vi "Build SendInput Struct.vi"(8 "error in (no error)":errorcluster, 10 "Data":u8[](array[numeric]), 11 "type":T1) -> (0 "error out":errorcluster, 3 "INPUT":u8[](array[numeric]))   [LabVIEW 2020, in "MacroAssert.lvlib" / "Win Util.lvlib"]
uses:
  Win Util.lvlib
  Input Type.ctl
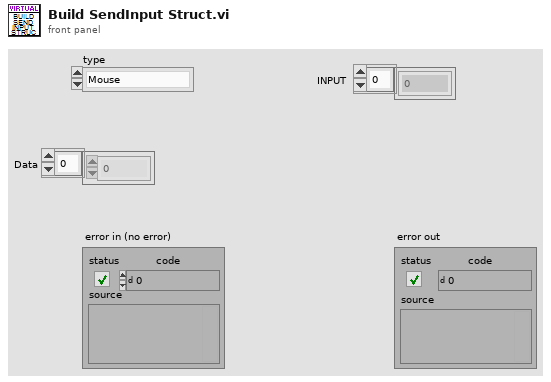
[diagram p1: front panel]
types:
  T1 = typedef "MacroAssert.lvlib/Win Util.lvlib/Input Type.ctl" = enum16{"Mouse", "Keyboard", "Hardware"}
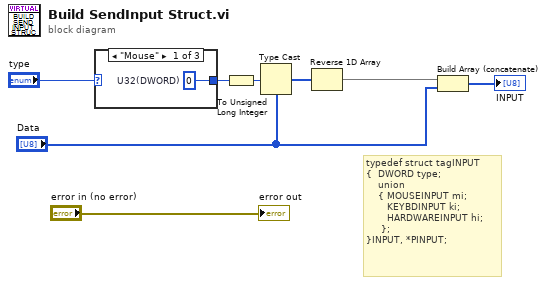
[diagram p0: block diagram]
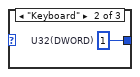
[diagram p2: hidden frame]
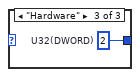
[diagram p3: hidden frame]
diagram:
  # "typedef struct tagINPUT\n{  DWORD type; \n    union\n    { MOUSEINPUT mi; \n       KEYBDINPUT ki;\n       HARDWAREINPUT hi;\n     };\n}INPUT, *PINPUT;"
  n1 = case shown="\"Mouse\"" "type" {
    tunnel: [w9 w10 w11] -> w8
    frame "Mouse" {
      w9 = u32 0  # U32(DWORD)
    }
    frame "Keyboard" {
      w10 = u32 1  # U32(DWORD)
    }
    frame "Hardware" {
      w11 = u32 2  # U32(DWORD)
    }
  }
  n2 = To Unsigned Long Integer(number=w8) -> (unsigned 32bit integer=w4:u32)
  n3 = Type Cast(type="Data", x=w4) -> (*(type *) &x=w5:u8[])
  n4 = Reverse 1D Array(array=w5) -> (reversed array=w3:u8[])
  n5 = Build Array (concatenate)(w3, "Data") -> (→"INPUT":u8[])
  "error out" <- "error in (no error)"
